vi "rotate complete.vi"(8 "error in (no error)":errorcluster caption="错误输入（无错误）", 9 "minimal error":dbl, 10 "current rotation":dbl[](array[numeric]), 11 "target rotation":dbl) -> (0 "error out":errorcluster caption="错误输出", 2 "rot complete":bool, 3 "rotation number":dbl)   [LabVIEW 2017]
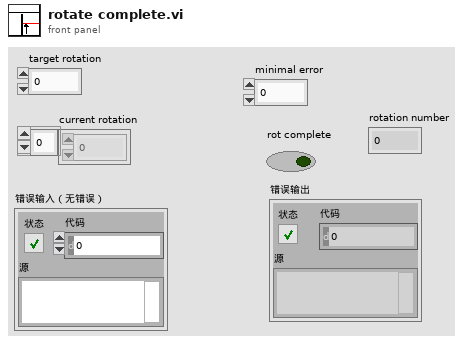
[diagram p1: front panel]
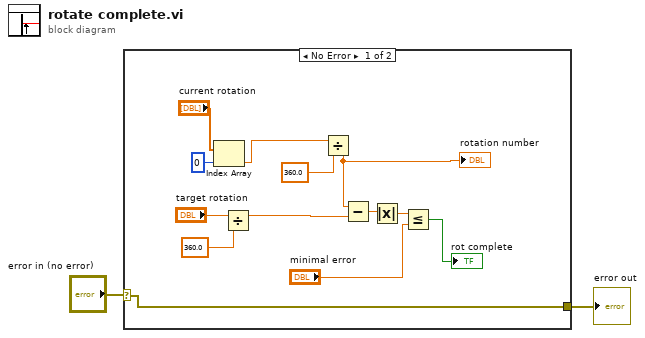
[diagram p0: block diagram]
diagram:
  n1 = case shown="No Error" "error in (no error)" {
    selector: "error in (no error)" -> [w3 w16]
    tunnel: [w3 w16] -> w1
    frame No Error {
      n2 = Index Array(array="current rotation", index=0 ("索引")) -> (element=w5:dbl)
      n3 = Divide(x="target rotation", y=360.0) -> (x/y=w8:dbl)
      n4 = Divide(x=w5, y=360.0) -> (x/y=w4:dbl)
      "rotation number" <- w4
      n5 = Subtract(x=w4, y=w8) -> (x-y=w15:dbl)
      n6 = Absolute Value(x=w15) -> (abs(x)=w11:dbl)
      n7 = Less Or Equal?(x=w11, y="minimal error") -> (x <= y?=→"rot complete":bool)
    }
    frame Error {
    }
  }
  "error out" <- w1
